vi "Host_Automate_Full_Timing_Study.vi"() -> ()   [LabVIEW 2021]
panel:
  out "Elasped Time (h:m:s)":string caption="Result"
  out "Experiment progress":u8(slide) scale=0.0..300.0
  out "Current test":T1
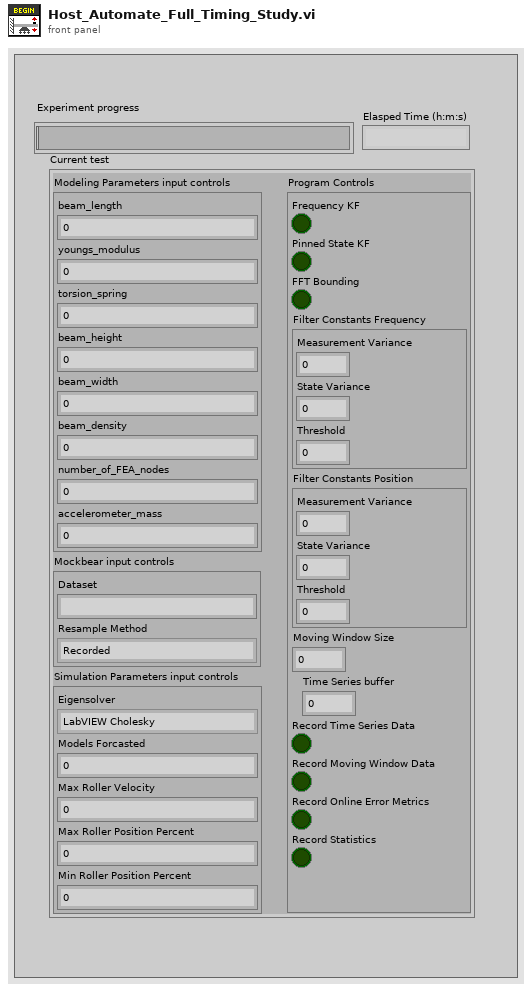
[diagram p1: front panel]
types:
  T1 = cluster{"Modeling Parameters input controls":cluster{"beam_length":dbl, "youngs_modulus":dbl, "torsion_spring":dbl, "beam_height":dbl, "beam_width":dbl, "beam_density":dbl, "number_of_FEA_nodes":i32, "accelerometer_mass":dbl}, "Mockbear input controls":cluster{"Dataset":string, "Resample Method":enum16{"Recorded", "Auto Resample", "Custom Resample"}}, "Simulation Parameters input controls":cluster{"Eigensolver ":enum16{"LabVIEW Cholesky", "LabVIEW General", "LabVIEW Inverse", "LEMP"}, "Models Forcasted":i32, "Max Roller Velocity":dbl, "Max Roller Position Percent":dbl, "Min Roller Position Percent":dbl}, "Program Controls":cluster{"Frequency KF":bool, "Pinned State KF":bool, "FFT Bounding":bool, "Filter Constants Frequency":cluster{"Measurement Variance":dbl, "State Variance":dbl, "Threshold":dbl}, "Filter Constants Position":cluster{"Measurement Variance":dbl, "State Variance":dbl, "Threshold":dbl}, "Moving Window Size":i32, "Time Series buffer":dbl, "Record Time Series Data":bool, "Record Moving Window Data":bool, "Record Online Error Metrics ":bool, "Record Statistics":bool}}
  T2 = cluster{"beam_length":dbl, "youngs_modulus":dbl, "torsion_spring":dbl, "beam_height":dbl, "beam_width":dbl, "beam_density":dbl, "number_of_FEA_nodes":i32, "accelerometer_mass":dbl}
  T3 = cluster{"Frequency KF":bool, "Pinned State KF":bool, "FFT Bounding":bool, "Filter Constants Frequency":cluster{"Measurement Variance":dbl, "State Variance":dbl, "Threshold":dbl}, "Filter Constants Position":cluster{"Measurement Variance":dbl, "State Variance":dbl, "Threshold":dbl}, "Moving Window Size":i32, "Time Series buffer":dbl, "Record Time Series Data":bool, "Record Moving Window Data":bool, "Record Online Error Metrics ":bool, "Record Statistics":bool}
  T4 = cluster{"Eigensolver ":enum16{"LabVIEW Cholesky", "LabVIEW General", "LabVIEW Inverse", "LEMP"}, "Models Forcasted":i32, "Max Roller Velocity":dbl, "Max Roller Position Percent":dbl, "Min Roller Position Percent":dbl}
  T5 = cluster{"Dataset":string, "Resample Method":enum16{"Recorded", "Auto Resample", "Custom Resample"}}
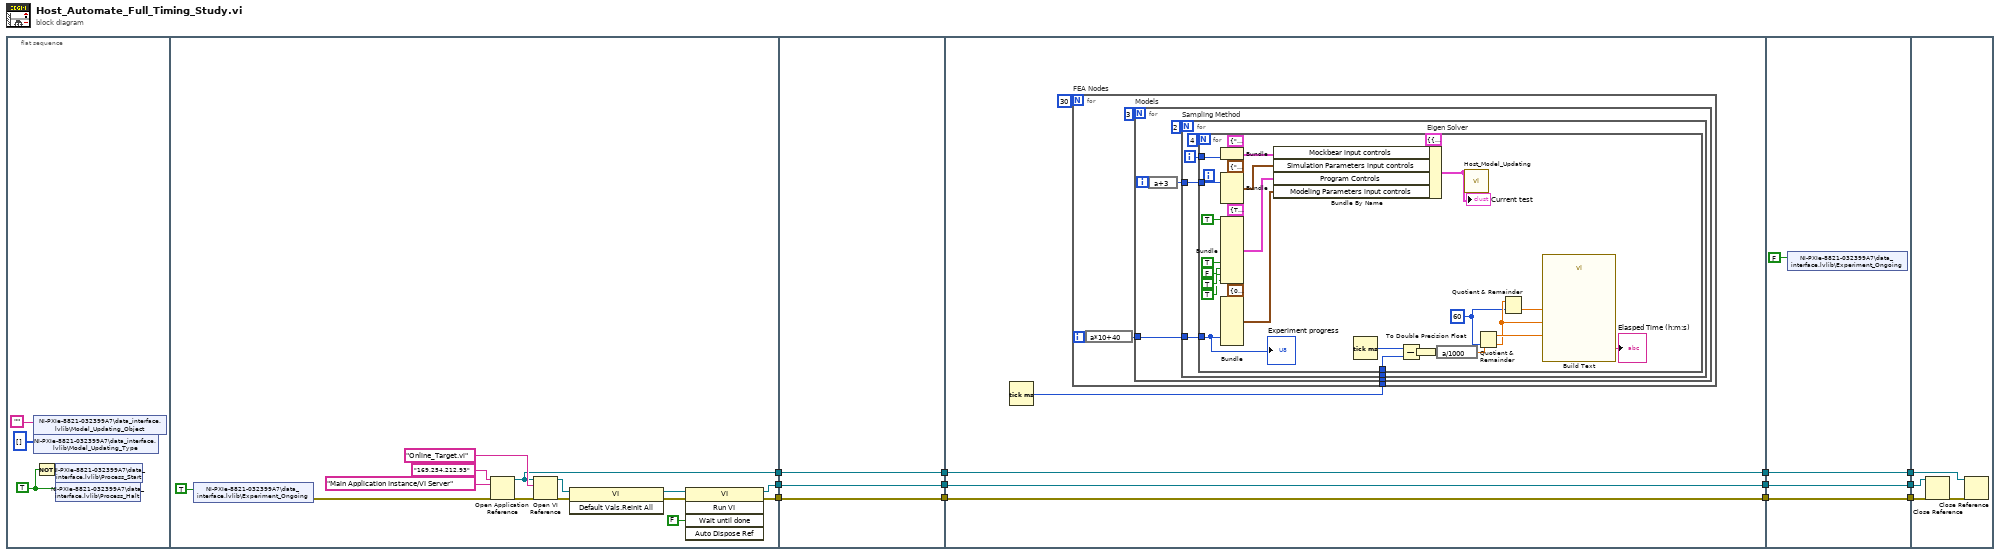
[diagram p0: block diagram]
diagram:
  n1 = flat-sequence {
    tunnel: [w23] -> w11
    tunnel: [w22] -> w9
    tunnel: [w21] -> w7
    tunnel: [w33] -> w12
    tunnel: w11 -> [w33]
    tunnel: [w32] -> w10
    tunnel: w9 -> [w32]
    tunnel: [w31] -> w8
    tunnel: w7 -> [w31]
    tunnel: [w36] -> w6
    tunnel: w12 -> [w36]
    tunnel: [w35] -> w4
    tunnel: w10 -> [w35]
    tunnel: [w34] -> w2
    tunnel: w8 -> [w34]
    tunnel: w6 -> [w84]
    tunnel: [w84] -> w5
    tunnel: w4 -> [w83]
    tunnel: [w83] -> w3
    tunnel: w2 -> [w82]
    tunnel: [w82] -> w1
    tunnel: w5 -> [w87]
    tunnel: w3 -> [w86]
    tunnel: w1 -> [w85]
    frame #0 {
      w14 = TRUE ("Process_Halt")
      n2 = shared-variable "NI-PXIe-8821-032399A7\\data_interface.lvlib\\Model_Updating_Object"("") -> ()  [unwired: 1 in, 1 out]
      n3 = shared-variable "NI-PXIe-8821-032399A7\\data_interface.lvlib\\Model_Updating_Type"(i16[] [] ("Model_Updating_Type")) -> ()  [unwired: 1 in, 1 out]
      n4 = Not(x=w14) -> (.not. x?=w13:bool)
      n5 = shared-variable "NI-PXIe-8821-032399A7\\data_interface.lvlib\\Process_Start"(w13) -> ()  [unwired: 1 in, 1 out]
      n6 = shared-variable "NI-PXIe-8821-032399A7\\data_interface.lvlib\\Process_Halt"(w14) -> ()  [unwired: 1 in, 1 out]
    }
    frame #1 {
      n7 = shared-variable "NI-PXIe-8821-032399A7\\data_interface.lvlib\\Experiment_Ongoing"(TRUE ("Experiment_Ongoing")) -> (error out=w19:errorcluster)  [unwired: 1 in]
      n8 = Open Application Reference(8:w19, 10:"Main Application Instance/VI Server", 11:"169.254.212.93") -> (0:w30:errorcluster, 3:w23:refnum<vi>)  [unwired: 1 in]
      n9 = Open VI Reference(application reference (local)=w23, vi path="Online_Target.vi", error in (no error)=w30) -> (vi reference=w18:refnum<vi>, error out=w26:errorcluster)  [unwired: 3 in]
      n10 = invoke class="VI" method="Default Vals.Reinit All"(reference=w18, error in=w26) -> (reference out=w25:refnum<vi>, error out=w24:errorcluster)  [unwired: 1 in, 1 out]
      n11 = invoke class="VI" method="Run VI"(reference=w25, error in=w24, "Wait until done"=FALSE ("Wait Until Done")) -> (reference out=w21:refnum<vi>, error out=w22:errorcluster)  [unwired: 2 in, 3 out]
    }
    frame #2 {
    }
    frame #3 {
      n12 = Tick Count (ms)() -> (millisecond timer value=w37:u32)
      n13 = for "FEA Nodes" {
        N: 30 -> [_]
        tunnel: w37 -> [w39]
        i -> [w41]
        n14 = expression code="a*10+40"(w41) -> (w40:i32)
        n15 = for "Models" {
          N: 3 -> [_]
          tunnel: w40 -> [w44]
          tunnel: w39 -> [w43]
          i -> [w46]
          n16 = expression code="a+3"(w46) -> (w45:i32)
          n17 = for "Sampling Method" {
            N: 2 -> [_]
            tunnel: w45 -> [w50]
            tunnel: w44 -> [w49]
            tunnel: w43 -> [w48]
            i -> [w51]
            n18 = for "Eigen Solver" {
              N: 4 -> [_]
              tunnel: w51 -> [w72]
              tunnel: w50 -> [w71]
              tunnel: w49 -> [w63]
              tunnel: w48 -> [w62]
              w55 = 60
              n19 = Bundle(cluster=T5 {"Dataset"="test7", "Resample Method"=enum."Auto Resample"} ("Mockbear input controls"), "Resample Method"=w72) -> (w73:T5)  [unwired: 1 in]
              n20 = Bundle(cluster=T4 {"Eigensolver "=enum."LEMP", "Models Forcasted"=5, "Max Roller Velocity"=3.32, "Max Roller Position Percent"=0.43, "Min Roller Position Percent"=0.155} ("Simulation Parameters input controls"), "Models Forcasted"=w71) -> (w74:T4)  [unwired: 4 in]
              n21 = Bundle(cluster=T3 {"Frequency KF"=TRUE, "Pinned State KF"=FALSE, "FFT Bounding"=FALSE, "Filter Constants Frequency"={"Measurement Variance"=0.4, "State Variance"=0.01, "Threshold"=1000000000.0}, "Filter Constants Position"={"Measurement Variance"=0.4, "State Variance"=0.9, "Threshold"=1000000000.0}, "Moving Window Size"=10, "Time Series buffer"=10000.0, "Record Time Series Data"=FALSE, "Record Moving Window Data"=FALSE, "Record Online Error Metrics "=TRUE, "Record Statistics"=TRUE} ("Program Controls"), "Frequency KF"=TRUE, "Record Time Series Data"=TRUE, "Record Moving Window Data"=FALSE, "Record Online Error Metrics"=TRUE, "Record Statistics"=TRUE) -> (w79:T3)  [unwired: 6 in]
              n22 = Bundle(cluster=T2 {"beam_length"=0.3525, "youngs_modulus"=209500000000.0, "torsion_spring"=0.0, "beam_height"=0.00635, "beam_width"=0.0508, "beam_density"=7900.0, "number_of_FEA_nodes"=40, "accelerometer_mass"=0.055} ("Modeling Parameters input controls"), "number_of_FEA_nodes"=w63) -> (w69:T2)  [unwired: 7 in]
              n23 = Bundle By Name(cluster=T1 {"Modeling Parameters input controls"={"beam_length"=0.3525, "youngs_modulus"=209500000000.0, "torsion_spring"=0.0, "beam_height"=0.00635, "beam_width"=0.0508, "beam_density"=7900.0, "number_of_FEA_nodes"=40, "accelerometer_mass"=0.055}, "Mockbear input controls"={"Dataset"="test7", "Resample Method"=enum."Auto Resample"}, "Simulation Parameters input controls"={"Eigensolver "=enum."LEMP", "Models Forcasted"=5, "Max Roller Velocity"=3.32, "Max Roller Position Percent"=0.43, "Min Roller Position Percent"=0.155}, "Program Controls"={"Frequency KF"=TRUE, "Pinned State KF"=FALSE, "FFT Bounding"=FALSE, "Filter Constants Frequency"={"Measurement Variance"=0.4, "State Variance"=0.01, "Threshold"=1000000000.0}, "Filter Constants Position"={"Measurement Variance"=0.4, "State Variance"=0.9, "Threshold"=1000000000.0}, "Moving Window Size"=10, "Time Series buffer"=10000.0, "Record Time Series Data"=FALSE, "Record Moving Window Data"=FALSE, "Record Online Error Metrics "=TRUE, "Record Statistics"=TRUE}} ("Setup Parameters and Controls"), "Mockbear input controls"=w73, "Simulation Parameters input controls"=w74, "Program Controls"=w79, "Modeling Parameters input controls"=w69) -> (w80:T1)
              "Current test" <- w80
              n24 = Tick Count (ms)() -> (millisecond timer value=w61:u32)
              n25 = Subtract(x=w61, y=w62) -> (x-y=w60:u32)
              n26 = To Double Precision Float(number=w60) -> (double precision float=w54:dbl)
              n27 = expression code="a/1000"(w54) -> (w57:dbl)
              n28 = call "Host_Model_Updating.vi"("Setup Parameters and Controls"=w80) -> ()  [unwired: 11 in]
              n29 = Quotient & Remainder(x=w57, y=w55) -> (x-y*floor(x/y)=w58:dbl, floor(x/y)=w56:dbl)
              n30 = Quotient & Remainder(x=w56, y=w55) -> (floor(x/y)=w59:dbl)  [unwired: 1 out]
              n31 = call "Build Text"("hours"=w59, "minutes"=w56, "seconds"=w58) -> ("Result"=→"Elasped Time (h:m:s)":string)  [unwired: 11 in, 1 out]
              "Experiment progress" <- w63
            }
          }
        }
      }
    }
    frame #4 {
      n32 = shared-variable "NI-PXIe-8821-032399A7\\data_interface.lvlib\\Experiment_Ongoing"(FALSE ("Experiment_Ongoing")) -> ()  [unwired: 1 in, 1 out]
    }
    frame #5 {
      n33 = Close Reference(reference=w85, error in (no error)=w86) -> (error out=w88:errorcluster)
      n34 = Close Reference(reference=w87, error in (no error)=w88) -> ()  [unwired: 1 out]
    }
  }
